vi "0-Write MDF.vi"(2 "error in":errorcluster, 3 "Waypoints List":T1) -> (0 "error out":errorcluster)   [LabVIEW 2011]
doc: "Saves a MDF (Mission Definition File) to be later opened by 0-Read MDF.vi. MDF contains mission data: currently only a list of waypoints. The file uses the LabVIEW XML Schema."
uses:
  0x2-OCU-Think Comm/0x2 Typedefs/Waypoints List.ctl
  0x2-OCU-Think Comm/0x2 Typedefs/ocuWaypoint.ctl
  0x2-OCU-Think Comm/0x2 Typedefs/waypointTypes.ctl
  2-Think/2 Typedefs/UTM Location.ctl
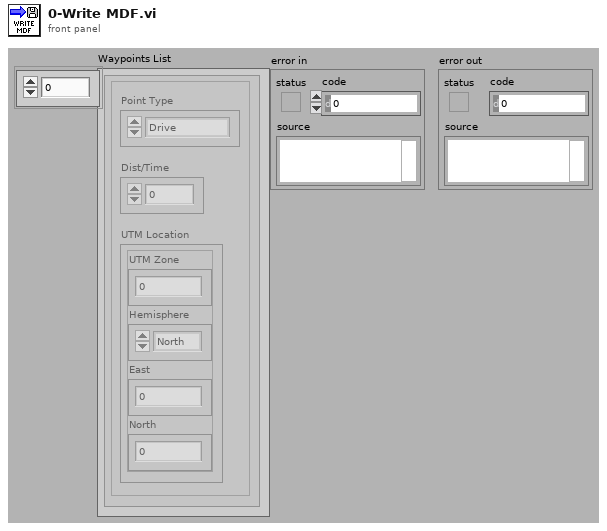
[diagram p1: front panel]
types:
  T1 = typedef "Waypoints List.ctl" = T2[]
  T2 = typedef "ocuWaypoint.ctl" = cluster{"Point Type":T3, "Dist/Time":dbl, "UTM Location":T4}
  T3 = typedef "waypointTypes.ctl" = enum16{"Drive", "Round Port", "Round Starboard", "Stay"}
  T4 = typedef "UTM Location.ctl" = cluster{"UTM Zone":dbl, "Hemisphere":enum16{"North", "South"}, "East":dbl, "North":dbl}
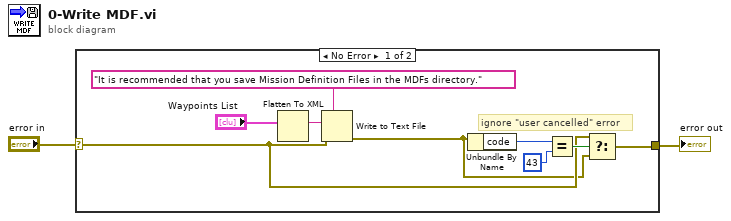
[diagram p0: block diagram]
diagram:
  n1 = case shown="No Error" "error in" {
    selector: "error in" -> [w5 w12]
    tunnel: [w3 w12] -> w1
    frame No Error {
      # "ignore \"user cancelled\" error"
      n2 = Flatten To XML(anything="Waypoints List") -> (xml string=w11:string)
      n3 = Write to Text File(prompt (Choose or enter file path)="It is recommended that you save Mission Definition Files in the MDFs directory.", text=w11, error in=w5) -> (error out=w4:errorcluster)  [unwired: 1 in, 2 out]
      n4 = Unbundle By Name(w4) -> ("code"=w8:i32)
      n5 = Equal?(x=w8, y=43 ("code")) -> (x = y?=w6:bool)
      n6 = Select(t=w5, s=w6, f=w4) -> (s? t:f=w3:errorcluster)
    }
    frame Error {
    }
  }
  "error out" <- w1
